vi "Function_save_conf_tomicro.vi"(6 "Class TCP in":T1, 7 "Saved configuration?":bool, 8 "error in (no error)":errorcluster, 10 "CmbBox Refnum in":refnum<vi>, 11 "ComboBox in":refnum<vi>) -> (0 "error out":errorcluster, 1 "Class TCP out":T1, 2 "Save conf?":bool, 3 "Connected?":bool, 5 "NB_CSs":i32)   [LabVIEW 2021]
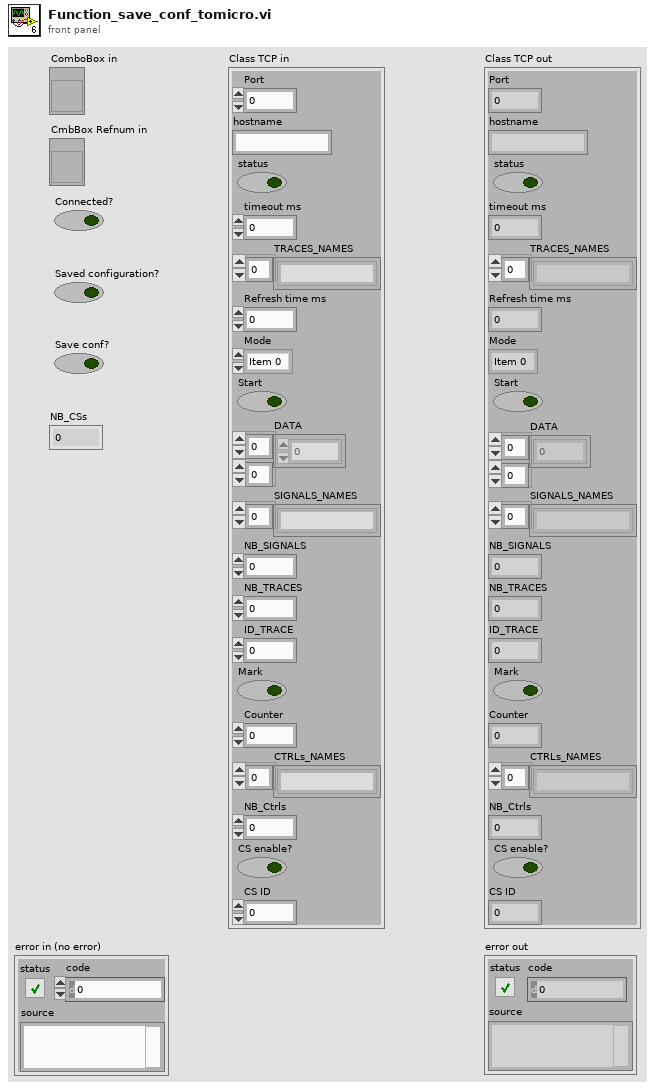
[diagram p1: front panel]
types:
  T1 = cluster{"Port":i32, "hostname":string, "status":bool, "timeout ms":i32, "TRACES_NAMES":string[], "Refresh time ms":i32, "Mode":enum32{"Item 0", "Item 1"}, "Start":bool, "DATA":sgl[][], "SIGNALS_NAMES":string[], "NB_SIGNALS":i32, "NB_TRACES":i32, "ID_TRACE":i32, "Mark":bool, "Counter":i32, "CTRLs_NAMES":string[], "NB_Ctrls":i32, "CS enable?":bool, "CS ID":i32}
  T2 = cluster{"timeout ms":i32, "remote port":u16, "Address":string}
  T3 = cluster{"SIZE":i32, " TRACE DATA":sgl[], "TRACE_SIZE":i32, "NB_TRACES":i32, "NB_TRACED_SIGNALS":i32, "NAMES TRACED SIGNALS":string[], "NAMES TRACES":string[], "CS STATUS":i32, "NB_CSs":i32, "NAMES CSs":string[], "DATA (M)":sgl[], "CMD":i32}
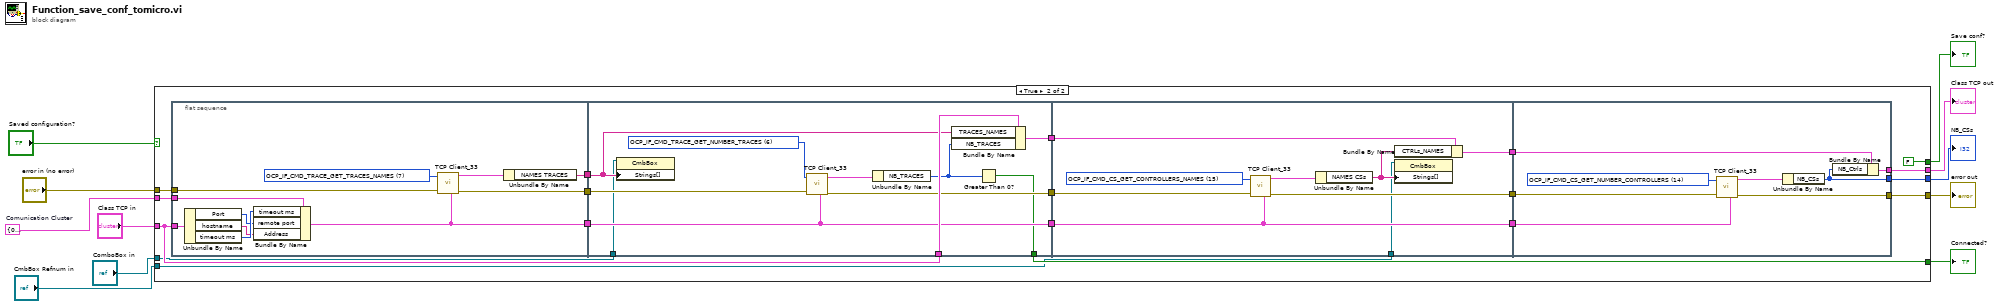
[diagram p0: block diagram]
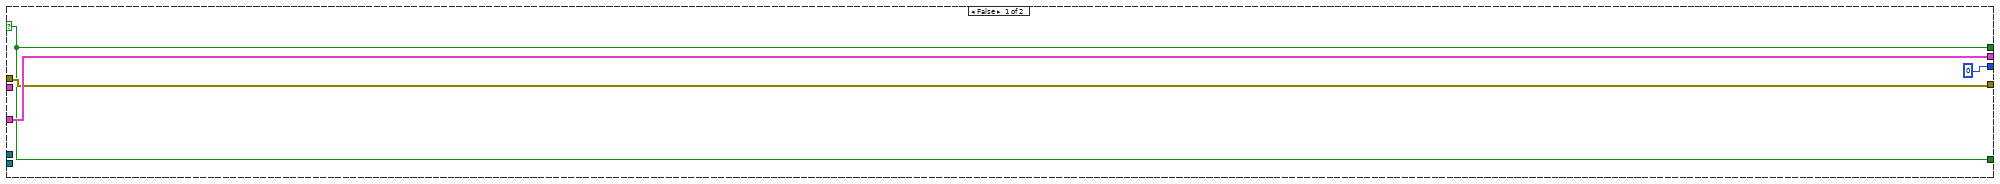
[diagram p2: hidden frame]
diagram:
  w8 = T2 {"timeout ms"=0, "remote port"=0, "Address"=""}  # Comunication Cluster
  n1 = case shown="True" "Saved configuration?" {
    selector: "Saved configuration?" -> [w13 _]
    tunnel: "error in (no error)" -> [w14 w22]
    tunnel: [w13 FALSE] -> w5
    tunnel: "Class TCP in" -> [w15 w33]
    tunnel: [w15 w32] -> w7
    tunnel: w8 -> [_ w21]
    tunnel: [w14 w20] -> w9
    tunnel: [w13 w19] -> w10
    tunnel: [0 ("NB_CSs") w18] -> w11
    tunnel: "ComboBox in" -> [_ w17]
    tunnel: "CmbBox Refnum in" -> [_ w16]
    frame False {
    }
    frame True {
      n2 = flat-sequence {
        tunnel: w33 -> [w45]
        tunnel: [w39] -> w31
        tunnel: [w38] -> w30
        tunnel: [w37] -> w29
        tunnel: w22 -> [w36]
        tunnel: w21 -> [w35]
        tunnel: w33 -> [w56]
        tunnel: w31 -> [w54]
        tunnel: w30 -> [w53]
        tunnel: w29 -> [w49]
        tunnel: [w55] -> w28
        tunnel: [w50] -> w26
        tunnel: [w49] -> w25
        tunnel: [w47] -> w19
        tunnel: w17 -> [w46]
        tunnel: w28 -> [w65]
        tunnel: [w59] -> w27
        tunnel: w26 -> [w64]
        tunnel: w25 -> [w61]
        tunnel: [w62] -> w24
        tunnel: [w61] -> w23
        tunnel: w16 -> [w57]
        tunnel: [w69] -> w32
        tunnel: w27 -> [w73]
        tunnel: w24 -> [w72]
        tunnel: w23 -> [w71]
        tunnel: [w67] -> w20
        tunnel: [w66] -> w18
        frame #0 {
          w44 = 7 items=["OCP_IF_CMD_TRACE_READ", "OCP_IF_CMD_TRACE_RESET", "OCP_IF_CMD_TRACE_GET_SIZE", "OCP_IF_CMD_TRACE_SET_SIZE", "OCP_IF_CMD_TRACE_GET_NUMBER_SIGNALS", "OCP_IF_CMD_TRACE_GET_SIGNALS_NAMES", "OCP_IF_CMD_TRACE_GET_NUMBER_TRACES", "OCP_IF_CMD_TRACE_GET_TRACES_NAMES", "OCP_IF_CMD_TRACE_GET_ADDRESS", "OCP_IF_CMD_CS_STATUS", "OCP_IF_CMD_CS_ENABLE", "OCP_IF_CMD_CS_DISABLE", "OCP_IF_CMD_CS_CONTROLLER_IF", "OCP_IF_CMD_CS_HARDWARE_IF", "OCP_IF_CMD_CS_GET_NUMBER_CONTROLLERS", "OCP_IF_CMD_CS_GET_CONTROLLERS_NAMES", "OCP_IF_CMD_PLATFORM_ID", "OCP_IF_CMD_PLATFORM_IF", "OCP_IF_CMD_OPIL_UPDATE_MEASUREMENTS", "OCP_IF_CMD_OPIL_UPDATE_SIM_DATA", "OCP_IF_CMD_OPIL_RUN_CONTROL", "OCP_IF_CMD_OPIL_INITIALIZE_CONTROL", "OCP_IF_CMD_OPIL_GET_CONTROL", "OCP_IF_CMD_OPIL_GET_CONTROLLER_DATA", "OCP_IF_CMD_END"] ("CMD")
          n3 = Unbundle By Name(w45) -> ("Port"=w41:i32, "hostname"=w40:string, "timeout ms"=w42:i32)
          n4 = Bundle By Name(cluster=w35, "timeout ms"=w42, "remote port"=w41, "Address"=w40) -> (w37:T2)
          n5 = call "TCP Client_33.vi"("CMD"=w44, "error in (no error)"=w36, "Comunication Cluster"=w37) -> ("Output cluster"=w43:T3, "error out"=w38:errorcluster)  [unwired: 5 in, 1 out]
          n6 = Unbundle By Name(w43) -> ("NAMES TRACES"=w39:string[])
        }
        frame #1 {
          w52 = 6 items=["OCP_IF_CMD_TRACE_READ", "OCP_IF_CMD_TRACE_RESET", "OCP_IF_CMD_TRACE_GET_SIZE", "OCP_IF_CMD_TRACE_SET_SIZE", "OCP_IF_CMD_TRACE_GET_NUMBER_SIGNALS", "OCP_IF_CMD_TRACE_GET_SIGNALS_NAMES", "OCP_IF_CMD_TRACE_GET_NUMBER_TRACES", "OCP_IF_CMD_TRACE_GET_TRACES_NAMES", "OCP_IF_CMD_TRACE_GET_ADDRESS", "OCP_IF_CMD_CS_STATUS", "OCP_IF_CMD_CS_ENABLE", "OCP_IF_CMD_CS_DISABLE", "OCP_IF_CMD_CS_CONTROLLER_IF", "OCP_IF_CMD_CS_HARDWARE_IF", "OCP_IF_CMD_CS_GET_NUMBER_CONTROLLERS", "OCP_IF_CMD_CS_GET_CONTROLLERS_NAMES", "OCP_IF_CMD_PLATFORM_ID", "OCP_IF_CMD_PLATFORM_IF", "OCP_IF_CMD_OPIL_UPDATE_MEASUREMENTS", "OCP_IF_CMD_OPIL_UPDATE_SIM_DATA", "OCP_IF_CMD_OPIL_RUN_CONTROL", "OCP_IF_CMD_OPIL_INITIALIZE_CONTROL", "OCP_IF_CMD_OPIL_GET_CONTROL", "OCP_IF_CMD_OPIL_GET_CONTROLLER_DATA", "OCP_IF_CMD_END"] ("CMD")
          n7 = property on="Property Node" class="CmbBox"(reference=w46, "Strings[]"=w54) -> ()  [unwired: 1 in, 2 out]
          n8 = call "TCP Client_33.vi"("CMD"=w52, "error in (no error)"=w53, "Comunication Cluster"=w49) -> ("Output cluster"=w51:T3, "error out"=w50:errorcluster)  [unwired: 5 in, 1 out]
          n9 = Unbundle By Name(w51) -> ("NB_TRACES"=w48:i32)
          n10 = Bundle By Name(cluster=w56, "TRACES_NAMES"=w54, "NB_TRACES"=w48) -> (w55:T1)
          n11 = Greater Than 0?(x=w48) -> (x > 0?=w47:bool)
        }
        frame #2 {
          w63 = 15 items=["OCP_IF_CMD_TRACE_READ", "OCP_IF_CMD_TRACE_RESET", "OCP_IF_CMD_TRACE_GET_SIZE", "OCP_IF_CMD_TRACE_SET_SIZE", "OCP_IF_CMD_TRACE_GET_NUMBER_SIGNALS", "OCP_IF_CMD_TRACE_GET_SIGNALS_NAMES", "OCP_IF_CMD_TRACE_GET_NUMBER_TRACES", "OCP_IF_CMD_TRACE_GET_TRACES_NAMES", "OCP_IF_CMD_TRACE_GET_ADDRESS", "OCP_IF_CMD_CS_STATUS", "OCP_IF_CMD_CS_ENABLE", "OCP_IF_CMD_CS_DISABLE", "OCP_IF_CMD_CS_CONTROLLER_IF", "OCP_IF_CMD_CS_HARDWARE_IF", "OCP_IF_CMD_CS_GET_NUMBER_CONTROLLERS", "OCP_IF_CMD_CS_GET_CONTROLLERS_NAMES", "OCP_IF_CMD_PLATFORM_ID", "OCP_IF_CMD_PLATFORM_IF", "OCP_IF_CMD_OPIL_UPDATE_MEASUREMENTS", "OCP_IF_CMD_OPIL_UPDATE_SIM_DATA", "OCP_IF_CMD_OPIL_RUN_CONTROL", "OCP_IF_CMD_OPIL_INITIALIZE_CONTROL", "OCP_IF_CMD_OPIL_GET_CONTROL", "OCP_IF_CMD_OPIL_GET_CONTROLLER_DATA", "OCP_IF_CMD_END"] ("CMD")
          n12 = call "TCP Client_33.vi"("CMD"=w63, "error in (no error)"=w64, "Comunication Cluster"=w61) -> ("Output cluster"=w60:T3, "error out"=w62:errorcluster)  [unwired: 5 in, 1 out]
          n13 = Unbundle By Name(w60) -> ("NAMES CSs"=w58:string[])
          n14 = Bundle By Name(cluster=w65, "CTRLs_NAMES"=w58) -> (w59:T1)
          n15 = property on="Property Node" class="CmbBox"(reference=w57, "Strings[]"=w58) -> ()  [unwired: 1 in, 2 out]
        }
        frame #3 {
          w70 = 14 items=["OCP_IF_CMD_TRACE_READ", "OCP_IF_CMD_TRACE_RESET", "OCP_IF_CMD_TRACE_GET_SIZE", "OCP_IF_CMD_TRACE_SET_SIZE", "OCP_IF_CMD_TRACE_GET_NUMBER_SIGNALS", "OCP_IF_CMD_TRACE_GET_SIGNALS_NAMES", "OCP_IF_CMD_TRACE_GET_NUMBER_TRACES", "OCP_IF_CMD_TRACE_GET_TRACES_NAMES", "OCP_IF_CMD_TRACE_GET_ADDRESS", "OCP_IF_CMD_CS_STATUS", "OCP_IF_CMD_CS_ENABLE", "OCP_IF_CMD_CS_DISABLE", "OCP_IF_CMD_CS_CONTROLLER_IF", "OCP_IF_CMD_CS_HARDWARE_IF", "OCP_IF_CMD_CS_GET_NUMBER_CONTROLLERS", "OCP_IF_CMD_CS_GET_CONTROLLERS_NAMES", "OCP_IF_CMD_PLATFORM_ID", "OCP_IF_CMD_PLATFORM_IF", "OCP_IF_CMD_OPIL_UPDATE_MEASUREMENTS", "OCP_IF_CMD_OPIL_UPDATE_SIM_DATA", "OCP_IF_CMD_OPIL_RUN_CONTROL", "OCP_IF_CMD_OPIL_INITIALIZE_CONTROL", "OCP_IF_CMD_OPIL_GET_CONTROL", "OCP_IF_CMD_OPIL_GET_CONTROLLER_DATA", "OCP_IF_CMD_END"] ("CMD")
          n16 = call "TCP Client_33.vi"("CMD"=w70, "error in (no error)"=w72, "Comunication Cluster"=w71) -> ("Output cluster"=w68:T3, "error out"=w67:errorcluster)  [unwired: 5 in, 1 out]
          n17 = Unbundle By Name(w68) -> ("NB_CSs"=w66:i32)
          n18 = Bundle By Name(cluster=w73, "NB_Ctrls"=w66) -> (w69:T1)
        }
      }
    }
  }
  "NB_CSs" <- w11
  "Connected?" <- w10
  "error out" <- w9
  "Class TCP out" <- w7
  "Save conf?" <- w5
